vi "Numerical Derivative.vi"(11 "Output Cluster":T1) -> (3 "Cluster":cluster{"Array Without Endpoints":dbl[], dbl[]})   [LabVIEW 2017]
uses:
  <vilib>/imath/engines/lvmath2/RunTimeEngine/Managers/WorkSpace/UID Generator.vi
  <vilib>/imath/engines/lvmath2/RunTimeEngine/RunTimeType/NIMS_RunTimeType_From StrictType (excl LVString).vi
  <instcachedir>/0/NIMS_RunTimeType_From StrictType (excl LVString)_1019F277F0A747EDBCA0F6C52CA54500.lvgen/NIMS_RunTimeType_From StrictType (excl LVString)_1019F277F0A747EDBCA0F6C52CA54500_000.vi
  <vilib>/imath/engines/lvmath2/RunTimeEngine/LocalVariableDefStatement/MC_LocalVariableDefStatement_Display.vi
  <vilib>/imath/engines/lvmath2/RunTimeEngine/Managers/SymbolTable/Clear UID.vi
  <vilib>/imath/engines/lvmath2/RunTimeEngine/NodeEndStatement/NIMS_NodeEndStatement_Output.vi
  <instcachedir>/0/NIMS_NodeEndStatement_Output_53EC0D466D134D7ABD903AC30B43404B.lvgen/NIMS_NodeEndStatement_Output_53EC0D466D134D7ABD903AC30B43404B_001.vi
  <vilib>/imath/engines/lvmath2/RunTimeEngine/ErrorHandling/NIMS_Finalize Error.vi
  <vilib>/imath/engines/lvmath2/RunTimeEngine/Managers/SymbolTable/NIMS_WorkSpace.lvlib
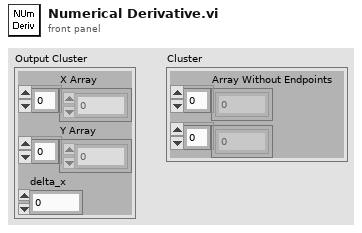
[diagram p1: front panel]
types:
  T1 = cluster{"X Array":dbl[], "Y Array":dbl[], "delta_x":dbl}
  T2 = cluster{"Sliced-off Array":dbl[], "Index-One Element":dbl, "Index Zero Element":dbl}
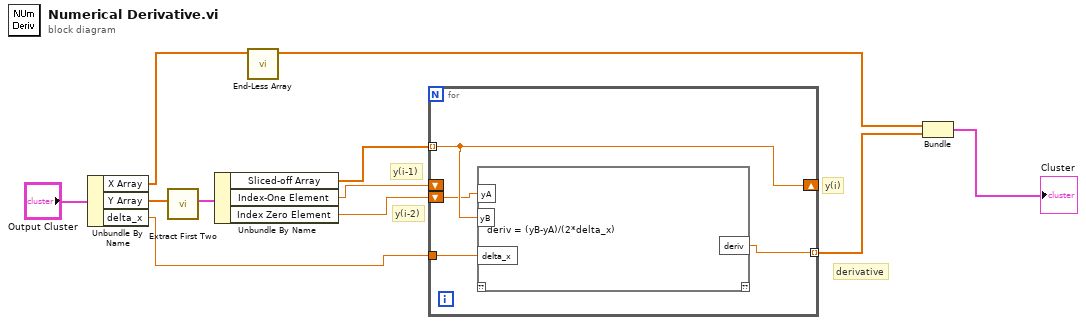
[diagram p0: block diagram]
diagram:
  # "derivative"
  # "y(i-2)"
  # "y(i-1)"
  # "y(i)"
  n1 = Unbundle By Name("Output Cluster") -> ("X Array"=w8:dbl[], "Y Array"=w2:dbl[], "delta_x"=w4:dbl)
  n2 = call "Extract First Two.vi"("Array"=w2) -> ("Output Cluster"=w3:T2)  [unwired: 10 in]
  n3 = Unbundle By Name(w3) -> ("Sliced-off Array"=w5:dbl[], "Index-One Element"=w6:dbl, "Index Zero Element"=w7:dbl)
  n4 = call "End-Less Array.vi"("Array"=w8) -> ("Array Without Endpoints"=w10:dbl[])  [unwired: 10 in]
  n5 = for {
    shift-right: [w15] -> _
    shift-left: w6 -> [_]
    shift-left: w7 -> [w14]
    tunnel: w5 -> [w15] mode=indexing
    tunnel: w4 -> [w13]
    tunnel: [w12] -> w9 mode=indexing
    n6 = mathscript code="deriv = (yB-yA)/(2*delta_x)"("yA"=w14, "yB"=w15, "delta_x"=w13) -> ("deriv"=w12:dbl)  [unwired: 1 in, 1 out]
  }
  n7 = Bundle("Array Without Endpoints"=w10, w9) -> (→"Cluster":cluster{"Array Without Endpoints":dbl[], dbl[]})  [unwired: 1 in]
